vi "Read IO.vi"(8 "error in (no error)":errorcluster, 11 "DAQmx in":refnum<class "DAQmx.lvclass">) -> (0 "error out":errorcluster, 3 "DAQmx out":refnum<class "DAQmx.lvclass">)   [LabVIEW 2016, in "DAQmx.lvclass"]
uses:
  DAQmx.lvclass
  Parent/Hardware.lvclass
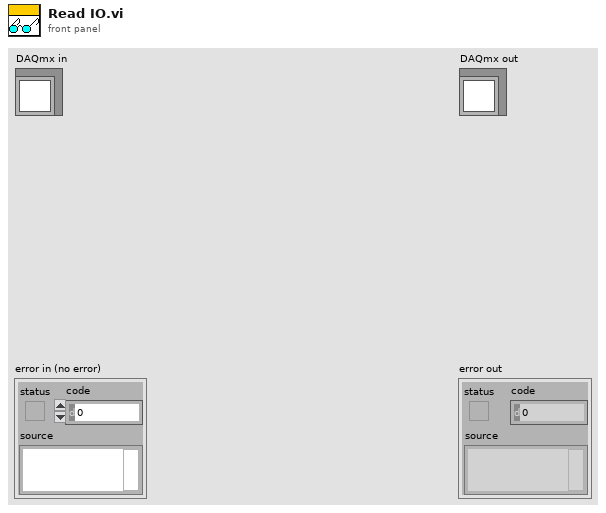
[diagram p1: front panel]
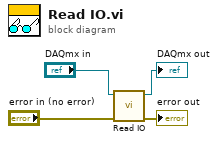
[diagram p0: block diagram]
diagram:
  n1 = call-parent "Read IO.vi"("error in (no error)"="error in (no error)", "Hardware in"="DAQmx in") -> ("error out"=→"error out":errorcluster, "Hardware out"=→"DAQmx out":refnum<class "DAQmx.lvclass">)  [unwired: 8 in]
